vi "HEWH Solenoid Output Set.vi"(6 "Debug":bool, 8 "Error In":errorcluster, 9 "HEWH MW100 Channel Numbers":T2="011", 10 "Outlet Valve":T1="OFF", 11 "VISA session":refnum<visa-resource-name>="MW100") -> (0 "Error Out":errorcluster, 3 "dup VISA session":refnum<visa-resource-name>)   [LabVIEW 2023]
uses:
  Type Definitions/HEWH MW100 Channel Numbers.ctl
  Type Definitions/HEWH Normally Open Valve Control.ctl
panel:
  out "Message":string
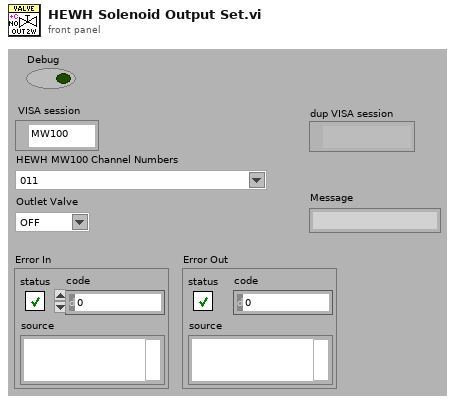
[diagram p1: front panel]
types:
  T1 = typedef "HEWH Normally Open Valve Control.ctl" = string
  T2 = typedef "HEWH MW100 Channel Numbers.ctl" = string
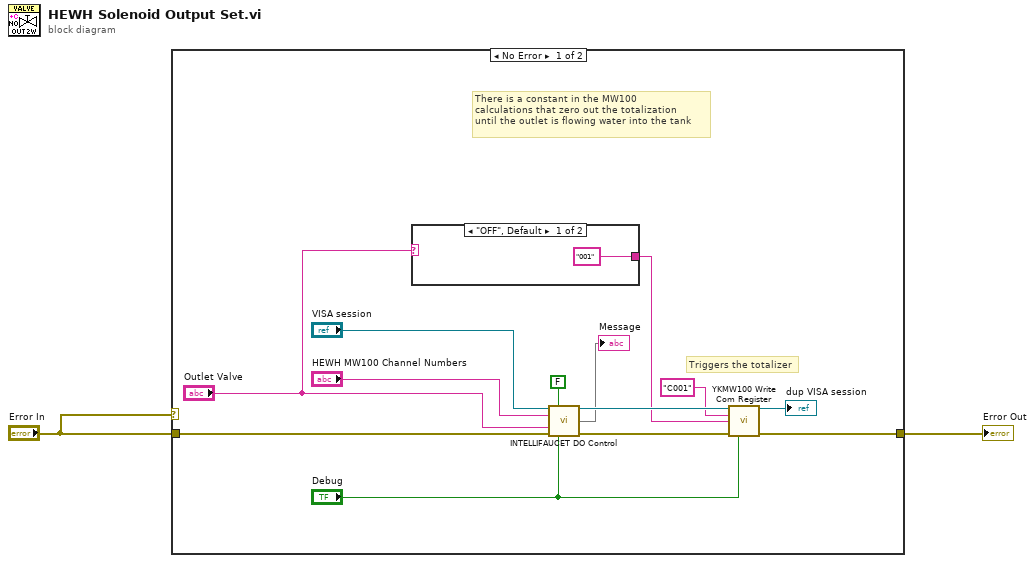
[diagram p0: block diagram]
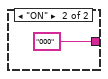
[diagram p2: hidden frame]
diagram:
  n1 = case shown="No Error" "Error In" {
    selector: "Error In" -> [_ w18]
    tunnel: "Error In" -> [w9 _]
    tunnel: [w8 w18] -> w2
    frame No Error {
      # "There is a constant in the MW100\ncalculations that zero out the totalization\nuntil the outlet is flowing water into the tank"
      # "Triggers the totalizer"
      n2 = case shown="\"OFF\", Default" "Outlet Valve" {
        tunnel: ["001" ("Channel") "000" ("Channel")] -> w10
        frame "OFF", Default {
        }
        frame "ON" {
        }
      }
      n3 = call "INTELLIFAUCET DO Control.vi"("VISA session"="VISA session", 1:FALSE ("Normally Closed Valve?"), "HEWH MW100 Channel Numbers"="HEWH MW100 Channel Numbers", 9:"Outlet Valve", "Error In"=w9, 12:"Debug") -> ("dup VISA session"=w12:refnum<visa-resource-name>, 8:→"Message", "error out"=w14:errorcluster)  [unwired: 7 in]
      n4 = call "YKMW100 Write Com Register.vi"("VISA session"=w12, "Channel"="C001", "Value"=w10, "error in (no error)"=w14, "Debug"="Debug") -> ("dup VISA session"=→"dup VISA session":refnum<visa-resource-name>, "error out"=w8:errorcluster)  [unwired: 9 in]
    }
    frame Error {
    }
  }
  "Error Out" <- w2
